vi "从机ID2.vi"(11 "ID号":u8) -> (1 "字符串":string, 3 "设备ID":dbl=255.0)   [LabVIEW 2012]
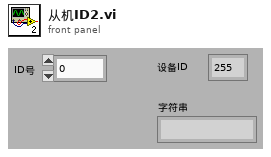
[diagram p1: front panel]
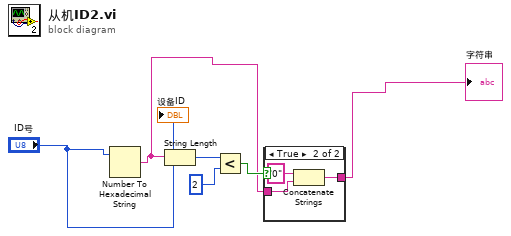
[diagram p0: block diagram]
diagram:
  n1 = Number To Hexadecimal String(2:"ID号") -> (0:w1:string)  [unwired: 1 out]
  n2 = String Length(string=w1) -> (length=w4:i32)
  n3 = Less?(x=w4, y=2) -> (x < y?=w2:bool)
  n4 = case shown="True" w2 {
    tunnel: [w7 w9] -> w6
    tunnel: w1 -> [w7 w8]
    frame False {
    }
    frame True {
      n5 = Concatenate Strings("0" ("字符串"), w8) -> (w9:string)
    }
  }
  "字符串" <- w6
  "设备ID" <- "ID号"
